vi "校准任务流程.vi"(9 "校准任务":T1[](array[typedef]), 10 "精度":dbl=4.0, 11 "模型":enum32{"线性", "多项式"}(ring)) -> ()   [LabVIEW 2016, in "斯坦道总氮.lvlib"]
uses:
  <userlib>/_OpenG.lib/array/array.llb/Remove Duplicates from 1D Array (U16)__ogtk.vi
panel:
  out "元素":T1
  out "执行列表":T2(ring)
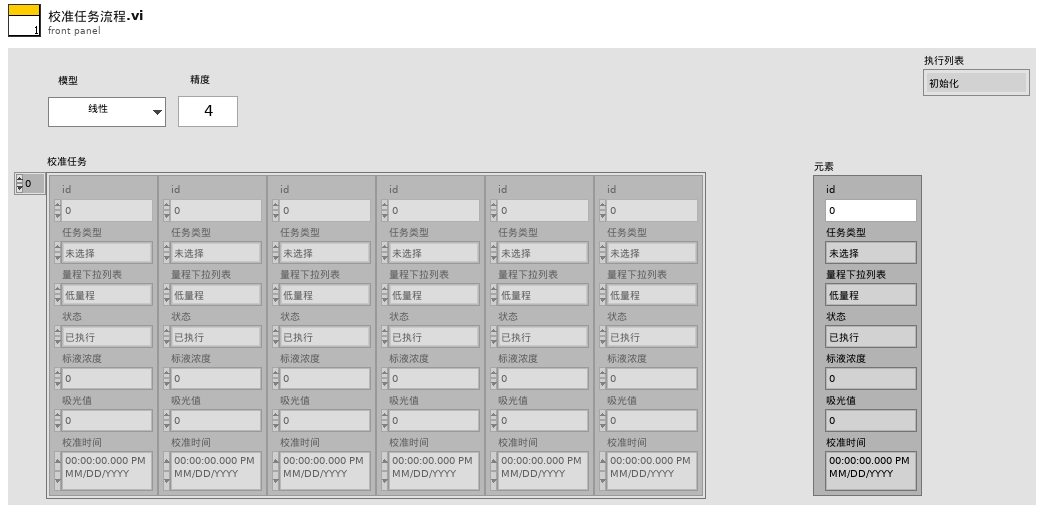
[diagram p1: front panel]
types:
  T1 = typedef "斯坦道总氮.lvlib/校准任务.ctl" = cluster{"id":u16, "任务类型":enum16{"未选择", "空白校准", "标样校准", "标样核查", "零点核查", "跨度核查"}, "量程下拉列表":enum16{"低量程", "高量程"}, "状态":enum16{"已执行", "待执行", "执行中", "停止"}, "标液浓度":dbl, "吸光值":dbl, "校准时间":timestamp}
  T2 = enum16{"初始化", "解析数据", "判断任务类型", "执行测试任务", "等待测试任务完成", "获取测试数据", "任务结束判定", "计算公式", "结束"}
  T3 = cluster{"时间标识":timestamp, "设备":string, "日志信息":string, "流程参数":string}
  T4 = cluster{"站号":u16, "量程切换":enum32{"H", "L", "AUTO"}, "控制命令":enum16{"启动测量", "标样核查", "零点核查", "跨度核查", "空白测试", "平行样测试", "加标回收", "空白校准", "标样校准", "初始化（清洗）", "停止测试", "仪器重启", "校时", "模式设置", "测量间隔设置"}, "模式设置":enum16{"待机", "连续模式", "周期模式", "定点模式", "受控模式", "手动模式"}, "测量间隔":u16}
  T5 = enum16{"启动测量", "标样核查", "零点核查", "跨度核查", "空白测试", "平行样测试", "加标回收", "空白校准", "标样校准", "初始化（清洗）", "停止测试", "仪器重启", "校时", "模式设置", "测量间隔设置"}
  T6 = cluster{"标液浓度1":dbl, "测量吸光度1":dbl, "样品1启用":bool, "标液浓度2":dbl, "测量吸光度2":dbl, "样品2启用":bool, "标液浓度3":dbl, "测量吸光度3":dbl, "样品3启用":bool, "标液浓度4":dbl, "测量吸光度4":dbl, "样品4启用":bool, "标液浓度5":dbl, "测量吸光度5":dbl, "样品5启用":bool, "模型":enum32{"线性", "多项式"}, "精度":dbl, "XY图":cluster{"X Values":dbl[], "Y Values":dbl[]}[], "拟合公式":string, "r^2":dbl, "标样一校准时间":timestamp, "标样二校准时间":timestamp, "标样三校准时间":timestamp, "标样四校准时间":timestamp, "标样五校准时间":timestamp, "二次方程":cluster{"c":dbl, "x":dbl, "x^2":dbl}, "标定时间":timestamp}
  T7 = cluster{"因子编码":u32, "单位":u16, "标样参考值":sgl, "水样数据时间":timestamp, "水样实测值":sgl, "水样数据标识":string, "标样数据时间":timestamp, "标样实测值":sgl, "标样数据标识":string, "空白数据时间":timestamp, "空白实测值":sgl, "空白数据标识":string, "零点核查数据时间":timestamp, "零点核查实测值":sgl, "零点核查数据标识":string, "跨度核查数据时间":timestamp, "跨度核查实测值":sgl, "跨度核查数据标识":string, "加标回收数据时间":timestamp, "加标回收实测值":sgl, "加标回收数据标识":string, "平行样数据时间":timestamp, "平行样实测值":sgl, "平行样数据标识":string, "F0":sgl, "F1":sgl, "F2":sgl, "F3":sgl, "F4":sgl, "F5":sgl, "F6":sgl, "F7":sgl, "温度":sgl, "湿度":sgl, "X值":sgl, "fidrange":u16, "X1值":sgl}
  T8 = cluster{"系统时间":timestamp, "工作状态":u16, "测量模式":enum16{"待机", "连续模式", "周期模式", "定点模式", "受控模式", "手动模式"}, "告警代码":u16, "故障代码":u16, "日志代码":u16, "软件版本":u16, "F0":sgl, "F1":sgl, "F2":sgl, "F3":sgl, "T":sgl, "H":sgl, "id":u16, "flowid":u16, "量程":u16, "总磷控温温度1":sgl, "营养盐控温温度2":sgl, "ADC":sgl, "结果值":sgl, "运行时间":u16, "步骤详情":string, "步骤流程":string}
  T9 = enum16{"未选择", "空白校准", "标样校准", "标样核查", "零点核查", "跨度核查"}
  T10 = cluster{"标液浓度1":dbl, "测量吸光度1":dbl, "样品1启用":bool, "标液浓度2":dbl, "测量吸光度2":dbl, "样品2启用":bool, "标液浓度3":dbl, "测量吸光度3":dbl, "样品3启用":bool, "标液浓度4":dbl, "测量吸光度4":dbl, "样品4启用":bool, "标液浓度5":dbl, "测量吸光度5":dbl, "样品5启用":bool, "模型":enum32{"线性", "多项式"}, "精度":dbl, "XY图":cluster{"X Values":dbl[], "Y Values":dbl[]}[], "拟合公式":string, "r^2":dbl, "标样一校准时间":timestamp, "标样二校准时间":timestamp, "标样三校准时间":timestamp, "标样四校准时间":timestamp, "标样五校准时间":timestamp, "二次方程":cluster{"c":dbl, "x":dbl, "x^2":dbl}, "标定时间":timestamp}[]
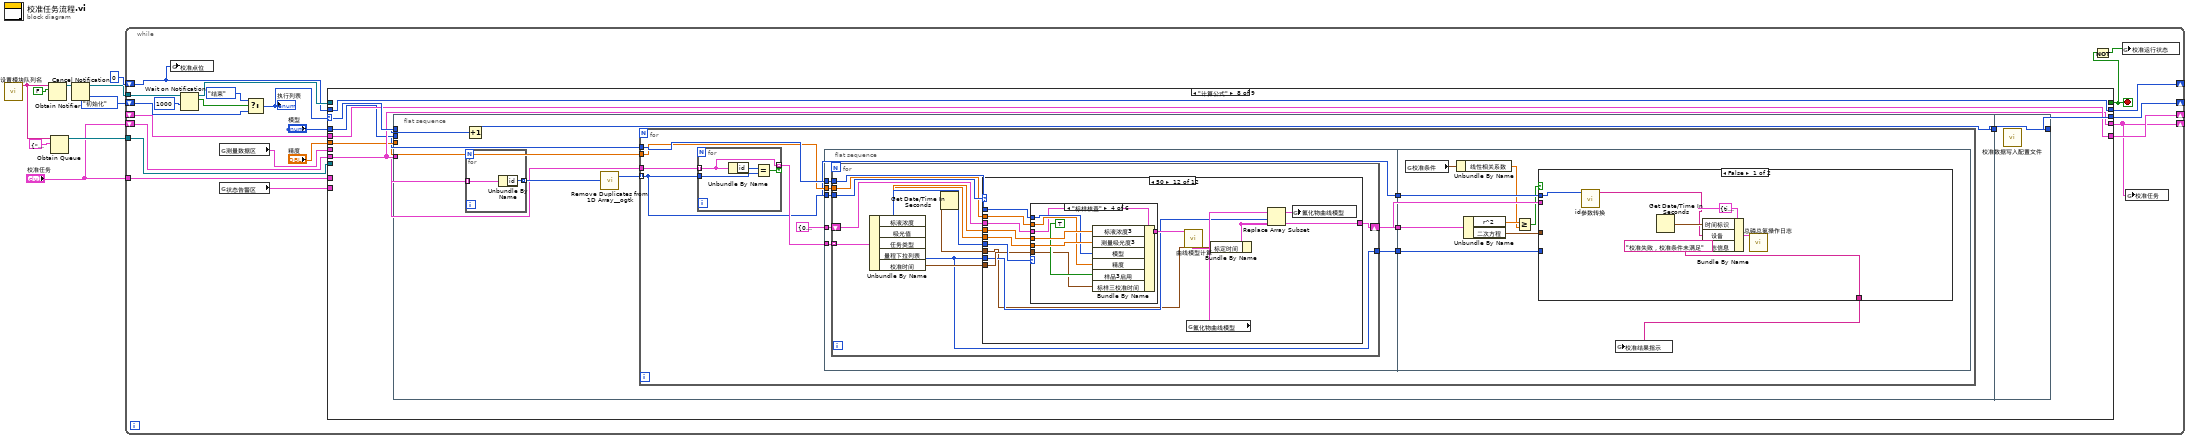
[diagram p0: block diagram]
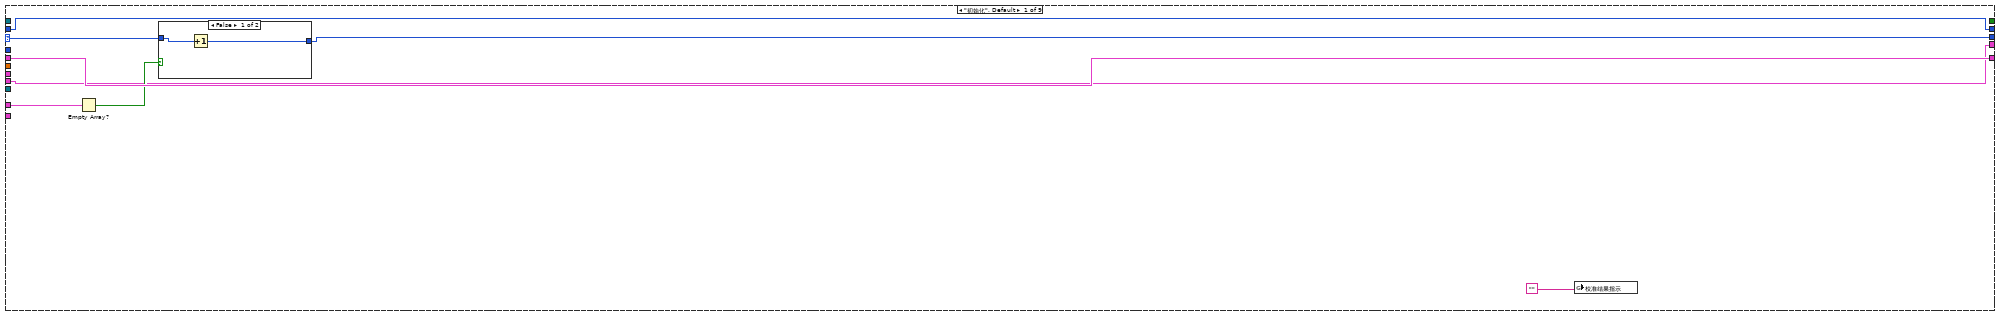
[diagram p2: hidden frame]
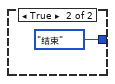
[diagram p3: hidden frame]
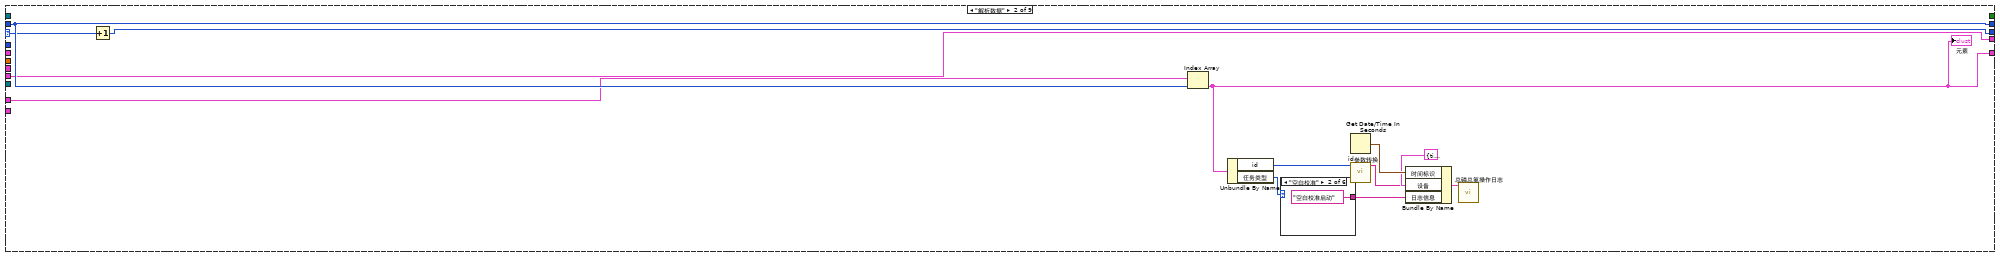
[diagram p4: hidden frame]
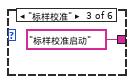
[diagram p6: hidden frame]
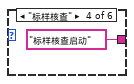
[diagram p7: hidden frame]
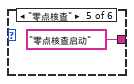
[diagram p8: hidden frame]
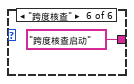
[diagram p9: hidden frame]
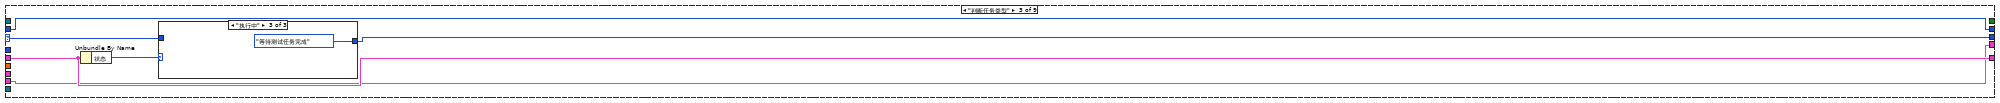
[diagram p10: hidden frame]
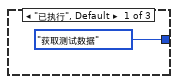
[diagram p11: hidden frame]
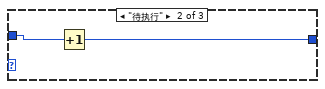
[diagram p12: hidden frame]
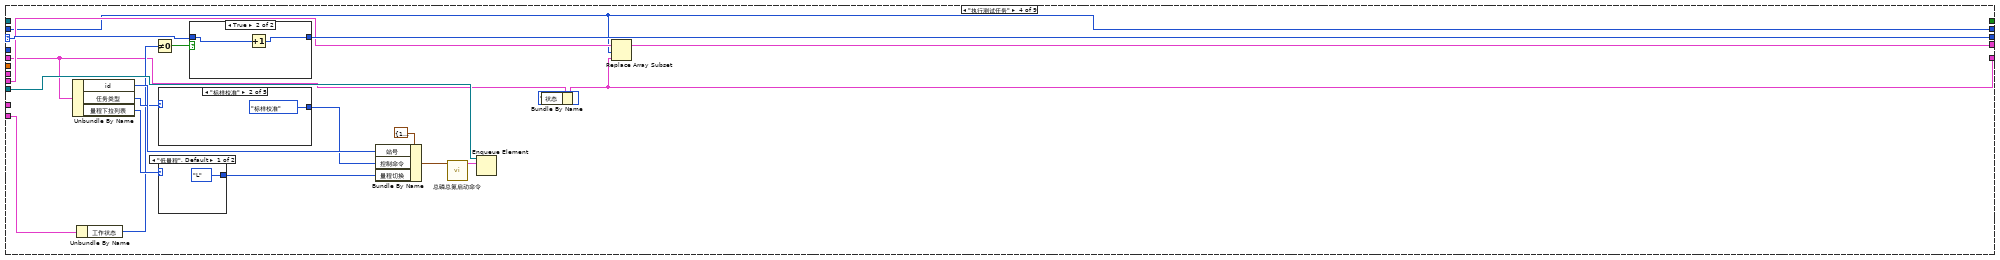
[diagram p13: hidden frame]
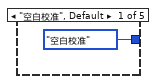
[diagram p15: hidden frame]
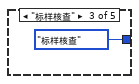
[diagram p16: hidden frame]
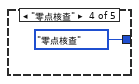
[diagram p17: hidden frame]
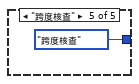
[diagram p18: hidden frame]
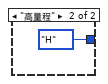
[diagram p19: hidden frame]
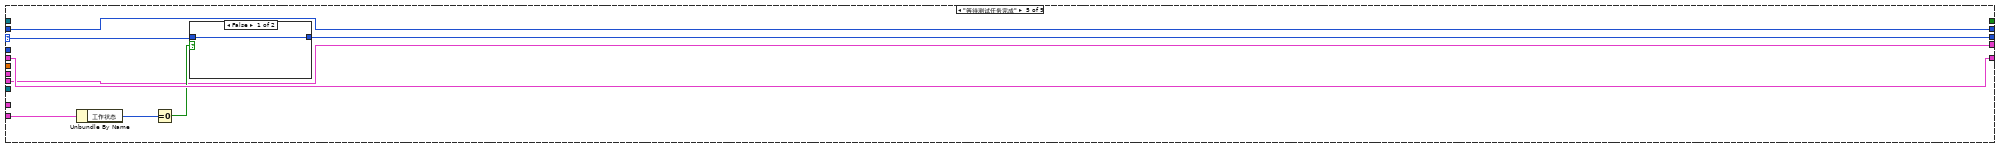
[diagram p20: hidden frame]
diagram:
  n1 = call "设置模块队列名.vi"() -> ("Msg"=w5:string)  [unwired: 5 in]
  n2 = Obtain Notifier(name (unnamed)=w5, notification data type=FALSE) -> (notifier out=w3:refnum<notifier>)  [unwired: 2 in, 2 out]
  n3 = Obtain Queue(name (unnamed)=w5, element data type=cluster{"命令":string, "data":variant} {"命令"="", "data"=variant}) -> (queue out=w4:refnum<queue>)  [unwired: 3 in, 2 out]
  n4 = Cancel Notification(0:w3) -> (8:w2:refnum<notifier>)  [unwired: 1 in, 2 out]
  n5 = while {
    shift-right: [w29] -> _
    shift-left: 0 -> [w11]
    shift-right: [w31] -> _
    shift-left: _ -> [w30]
    shift-right: [w28] -> _
    shift-left: T2."初始化" ("执行列表") -> [w17]
    tunnel: w4 -> [w27]
    tunnel: w2 -> [w26]
    tunnel: "校准任务" -> [w23]
    shift-right: [w10] -> _
    shift-left: "校准任务" -> [w22]
    stop <- w12 stop-if-true
    n6 = global write "VAR总磷总氮全局变量.vi" "校准点位"(w11) -> ()
    n7 = Wait on Notification(notifier=w26, timeout in ms (-1)=1000 ("超时毫秒(-1)")) -> (notifier out=w19:refnum<notifier>, notification=w18:bool)  [unwired: 2 in, 2 out]
    n8 = global read "VAR总磷总氮全局变量.vi" "测量数据区"() -> (w24:T7)
    n9 = global read "VAR总磷总氮全局变量.vi" "状态告警区"() -> (w25:T8)
    n10 = Select(t=T2."结束", s=w18, f=w17) -> (s? t:f=w16:T2)
    "执行列表" <- w16
    n11 = case shown="\"计算公式\"" w16 {
      selector: w16 -> [w37 w54 w63 w78 w104 w121 w152 w165 w859]
      tunnel: w11 -> [w38 w55 w65 w74 w107 w112 w153 w163 w857]
      tunnel: [w39 w46 w66 w71 w108 w116 w154 w162 w858] -> w31
      tunnel: w30 -> [w39 _ w66 w73 w108 w116 w154 w162 w858]
      tunnel: [w38 w55 w65 w74 w107 w112 w149 w163 w857] -> w29
      tunnel: [_ _ _ _ _ _ _ _ TRUE] -> w12
      tunnel: [w36 w53 w62 w77 w102 w120 w151 w164 w859] -> w28
      tunnel: w27 -> [_ _ _ w89 _ _ _ _ w854]
      tunnel: w19 -> [_ _ _ _ _ _ _ _ w853]
      tunnel: w25 -> [_ _ _ w81 w106 _ _ _ _]
      tunnel: w24 -> [_ _ _ _ _ w123 _ _ _]
      tunnel: w23 -> [w34 w52 _ _ _ _ w150 _ _]
      tunnel: [w33 w51 w61 w75 w101 w118 w146 w161 w855] -> w10
      tunnel: w22 -> [w33 w51 w61 w76 w101 w117 w146 w161 w855]
      tunnel: "模型" -> [_ _ _ _ _ _ _ w160 _]
      tunnel: "精度" -> [_ _ _ _ _ _ _ w159 _]
      frame "初始化", Default {
        n12 = Empty Array?(array=w34) -> (empty?=w35:bool)
        n13 = case shown="False" w35 {
          tunnel: w37 -> [w41 _]
          tunnel: [w40 T2."结束"] -> w36
          frame False {
            n14 = Increment(x=w41) -> (x+1=w40:T2)
          }
          frame True {
          }
        }
        n15 = global write "VAR总磷总氮全局变量.vi" "校准结果指示"("") -> ()
      }
      frame "解析数据" {
        n16 = Increment(x=w54) -> (x+1=w53:T2)
        n17 = Index Array(array=w52, index=w55) -> (element=w46:T1)
        "元素" <- w46
        n18 = Unbundle By Name(w46) -> ("id"=w45:u16, "任务类型"=w44:T9)
        n19 = case shown="\"空白校准\"" w44 {
          tunnel: [_ "空白校准启动" "标样校准启动" "标样核查启动" "零点核查启动" "跨度核查启动"] -> w43
          frame "未选择", Default {
          }
          frame "空白校准" {
          }
          frame "标样校准" {
          }
          frame "标样核查" {
          }
          frame "零点核查" {
          }
          frame "跨度核查" {
          }
        }
        n20 = Get Date/Time In Seconds() -> (seconds since 1Jan1904=w50:timestamp)
        n21 = call "id参数转换.vi"("id"=w45) -> ("table输出"=w47:string)  [unwired: 9 in, 1 out]
        n22 = Bundle By Name(cluster=T3 {"时间标识"=timestamp(0 s since 1904-01-01), "设备"="", "日志信息"="", "流程参数"=""} ("data in"), "时间标识"=w50, "设备"=w47, "日志信息"=w43) -> (w49:T3)
        n23 = call "总磷总氮操作日志.vi"("data in"=w49) -> ()  [unwired: 10 in, 1 out]
      }
      frame "判断任务类型" {
        n24 = Unbundle By Name(w66) -> ("状态"=w64:enum16{"已执行", "待执行", "执行中", "停止"})
        n25 = case shown="\"执行中\"" w64 {
          tunnel: w63 -> [_ w69 _]
          tunnel: [T2."获取测试数据" w68 T2."等待测试任务完成"] -> w62
          frame "已执行", Default {
          }
          frame "待执行" {
            n26 = Increment(x=w69) -> (x+1=w68:T2)
          }
          frame "执行中" {
          }
        }
      }
      frame "执行测试任务" {
        n27 = Unbundle By Name(w73) -> ("id"=w87:u16, "任务类型"=w86:T9, "量程下拉列表"=w85:enum16{"低量程", "高量程"})
        n28 = Unbundle By Name(w81) -> ("工作状态"=w80:u16)
        n29 = Not Equal To 0?(x=w80) -> (x != 0?=w79:bool)
        n30 = case shown="\"标样校准\"" w86 {
          tunnel: [T5."空白校准" ("控制命令") T5."标样校准" ("控制命令") T5."标样核查" ("控制命令") T5."零点核查" ("控制命令") T5."跨度核查" ("控制命令")] -> w84
          frame "空白校准", Default {
          }
          frame "标样校准" {
          }
          frame "标样核查" {
          }
          frame "零点核查" {
          }
          frame "跨度核查" {
          }
        }
        n31 = case shown="\"低量程\", Default" w85 {
          tunnel: [enum32{"H", "L", "AUTO"}."L" ("量程切换") enum32{"H", "L", "AUTO"}."H" ("量程切换")] -> w82
          frame "低量程", Default {
          }
          frame "高量程" {
          }
        }
        n32 = case shown="True" w79 {
          tunnel: w78 -> [w91 w93]
          tunnel: [w91 w92] -> w77
          frame False {
          }
          frame True {
            n33 = Increment(x=w93) -> (x+1=w92:T2)
          }
        }
        n34 = Bundle By Name(cluster=T4 {"站号"=1, "量程切换"=enum."AUTO", "控制命令"=enum."启动测量", "模式设置"=enum."待机", "测量间隔"=0} ("参数"), "站号"=w87, "控制命令"=w84, "量程切换"=w82) -> (w83:T4)
        n35 = call "总磷总氮启动命令.vi"("参数"=w83) -> ("启动命令"=w90:cluster{"命令":string, "data":variant})  [unwired: 10 in]
        n36 = Enqueue Element(queue=w89, element=w90) -> ()  [unwired: 2 in, 3 out]
        n37 = Bundle By Name(cluster=w73, "状态"=enum16{"已执行", "待执行", "执行中", "停止"}."执行中") -> (w71:T1)
        n38 = Replace Array Subset(array=w76, new element=w71, index=w74) -> (w75:T1[])
      }
      frame "等待测试任务完成" {
        n39 = Unbundle By Name(w106) -> ("工作状态"=w105:u16)
        n40 = Equal To 0?(x=w105) -> (x = 0?=w103:bool)
        n41 = case shown="False" w103 {
          tunnel: w104 -> [w109 w111]
          tunnel: [w109 w110] -> w102
          frame False {
          }
          frame True {
            n42 = Increment(x=w111) -> (x+1=w110:T2)
          }
        }
      }
      frame "获取测试数据" {
        n43 = Unbundle By Name(w116) -> ("任务类型"=w122:T9, "状态"=w115:enum16{"已执行", "待执行", "执行中", "停止"})
        n44 = Increment(x=w121) -> (x+1=w120:T2)
        n45 = case shown="\"已执行\", Default" w115 {
          tunnel: w123 -> [_ w130]
          tunnel: w122 -> [_ w129]
          tunnel: [w124 w126] -> w119
          tunnel: w116 -> [w124 w125]
          frame "已执行", Default {
          }
          frame "执行中" {
            n46 = case shown="\"标样校准\"" w129 {
              tunnel: w130 -> [w133 w136 w139 w142 w145]
              tunnel: [w132 w135 w138 w141 w144] -> w127
              tunnel: [w131 w134 w137 w140 w143] -> w128
              frame "空白校准", Default {
                n47 = Unbundle By Name(w133) -> ("空白数据时间"=w132:timestamp, "X值"=w131:sgl)
              }
              frame "标样校准" {
                n48 = Unbundle By Name(w136) -> ("标样数据时间"=w135:timestamp, "X值"=w134:sgl)
              }
              frame "标样核查" {
                n49 = Unbundle By Name(w139) -> ("标样数据时间"=w138:timestamp, "X值"=w137:sgl)
              }
              frame "零点核查" {
                n50 = Unbundle By Name(w142) -> ("零点核查数据时间"=w141:timestamp, "X值"=w140:sgl)
              }
              frame "跨度核查" {
                n51 = Unbundle By Name(w145) -> ("跨度核查数据时间"=w144:timestamp, "X值"=w143:sgl)
              }
            }
            n52 = Bundle By Name(cluster=w125, "校准时间"=w127, "吸光值"=w128) -> (w126:T1)
          }
        }
        n53 = Bundle By Name(cluster=w119, "状态"=enum16{"已执行", "待执行", "执行中", "停止"}."已执行") -> (w113:T1)
        n54 = Replace Array Subset(array=w117, new element=w113, index=w112) -> (w118:T1[])
      }
      frame "任务结束判定" {
        n55 = Array Size(array=w150) -> (size(s)=w148:i32)
        n56 = Increment(x=w153) -> (x+1=w149:i32)
        n57 = Greater Or Equal?(x=w149, y=w148) -> (x >= y?=w147:bool)
        n58 = case shown="False" w147 {
          tunnel: w152 -> [_ w157]
          tunnel: [T2."解析数据" w156] -> w151
          frame False {
          }
          frame True {
            n59 = Increment(x=w157) -> (x+1=w156:T2)
          }
        }
      }
      frame "计算公式" {
        n60 = flat-sequence {
          tunnel: w165 -> [w172]
          tunnel: w161 -> [w168]
          tunnel: w160 -> [w167]
          tunnel: w159 -> [w166]
          tunnel: [w171] -> w158
          tunnel: [w852] -> w164
          tunnel: w158 -> [w852]
          frame #0 {
            n61 = for {
              tunnel: w168 -> [w851] mode=indexing
              tunnel: [w850] -> w170 mode=indexing
              n62 = Unbundle By Name(w851) -> ("id"=w850:u16)
            }
            n63 = Increment(x=w172) -> (x+1=w171:T2)
            n64 = call-poly <userlib>:"Remove Duplicates from 1D Array__ogtk.vi"("Input Array"=w170) -> ("Output Array"=w169:u16[])  [unwired: 1 out]
            n65 = for {
              tunnel: w169 -> [w179] mode=indexing
              tunnel: w168 -> [w181]
              tunnel: w167 -> [w178]
              tunnel: w166 -> [w177]
              n66 = for {
                tunnel: w181 -> [w847] mode=indexing
                tunnel: w179 -> [w849]
                tunnel: [w847] -> w180 mode=indexing if=w848
                n67 = Unbundle By Name(w847) -> ("id"=w846:u16)
                n68 = Equal?(x=w846, y=w849) -> (x = y?=w848:bool)
              }
              n69 = flat-sequence {
                tunnel: w180 -> [w188]
                tunnel: w179 -> [w183]
                tunnel: w178 -> [w187]
                tunnel: w177 -> [w186]
                tunnel: T6 {"标液浓度1"=0.0, "测量吸光度1"=0.0, "样品1启用"=FALSE, "标液浓度2"=0.0, "测量吸光度2"=0.0, "样品2启用"=FALSE, "标液浓度3"=0.0, "测量吸光度3"=0.0, "样品3启用"=FALSE, "标液浓度4"=0.0, "测量吸光度4"=0.0, "样品4启用"=FALSE, "标液浓度5"=0.0, "测量吸光度5"=0.0, "样品5启用"=FALSE, "模型"=enum."线性", "精度"=0.0, "XY图"=[], "拟合公式"="", "r^2"=0.0, "标样一校准时间"=timestamp(0 s since 1904-01-01), "标样二校准时间"=timestamp(0 s since 1904-01-01), "标样三校准时间"=timestamp(0 s since 1904-01-01), "标样四校准时间"=timestamp(0 s since 1904-01-01), "标样五校准时间"=timestamp(0 s since 1904-01-01), "二次方程"={"c"=0.0, "x"=0.0, "x^2"=0.0}, "标定时间"=timestamp(0 s since 1904-01-01)} ("新元素/子数组") -> [w185]
                tunnel: [w184] -> w175
                tunnel: [w183] -> w174
                tunnel: [w182] -> w173
                tunnel: w175 -> [w812]
                tunnel: w174 -> [w814]
                tunnel: w173 -> [w813]
                frame #0 {
                  n70 = for {
                    tunnel: w188 -> [w200] mode=indexing
                    tunnel: w183 -> [w199]
                    tunnel: w187 -> [w195]
                    tunnel: w186 -> [w194]
                    shift-right: [w192] -> w184
                    shift-left: w185 -> [w193]
                    tunnel: [w190] -> w182
                    n71 = Unbundle By Name(w200) -> ("标液浓度"=w197:dbl, "吸光值"=w196:dbl, "任务类型"=w198:T9, "量程下拉列表"=w190:enum16{"低量程", "高量程"}, "校准时间"=w191:timestamp)
                    n72 = Get Date/Time In Seconds() -> (seconds since 1Jan1904=w189:timestamp)
                    n73 = case shown="50" w199 {
                      tunnel: w190 -> [_ w204 w261 w316 w372 w425 w479 w535 w591 w645 w700 w755]
                      tunnel: w198 -> [_ w215 w270 w325 w380 w435 w490 w545 w600 w655 w710 w765]
                      tunnel: w197 -> [_ w214 w269 w324 w379 w434 w489 w544 w599 w654 w709 w764]
                      tunnel: w196 -> [_ w213 w268 w323 w378 w433 w488 w543 w598 w653 w708 w763]
                      tunnel: w195 -> [_ w212 w267 w322 w377 w432 w487 w542 w597 w652 w707 w762]
                      tunnel: w194 -> [_ w211 w266 w321 w376 w431 w486 w541 w596 w651 w706 w761]
                      tunnel: w193 -> [w201 w210 w265 w320 w375 w430 w485 w540 w595 w650 w705 w760]
                      tunnel: [w201 w203 w258 w313 w368 w423 w478 w533 w588 w643 w698 w753] -> w192
                      tunnel: w191 -> [_ w209 w264 w319 w374 w429 w484 w539 w594 w649 w704 w759]
                      tunnel: w189 -> [_ w202 w257 w312 w367 w422 w477 w532 w587 w642 w697 w752]
                      frame 0, Default {
                      }
                      frame 1 {
                        n74 = case shown="\"未选择\", Default" w215 {
                          tunnel: w214 -> [_ w224 w232 w240 w248 w256]
                          tunnel: w213 -> [_ w223 w231 w239 w247 w255]
                          tunnel: w212 -> [_ w222 w230 w238 w246 w254]
                          tunnel: w211 -> [_ w221 w229 w237 w245 w253]
                          tunnel: w210 -> [w216 w219 w227 w235 w243 w251]
                          tunnel: [w216 w217 w226 w234 w242 w250] -> w206
                          tunnel: w209 -> [_ w218 w225 w233 w241 w249]
                          frame "未选择", Default {
                          }
                          frame "空白校准" {
                            n75 = Bundle By Name(cluster=w219, "标液浓度1"=w224, "测量吸光度1"=w223, "模型"=w222, "精度"=w221, "样品1启用"=TRUE, "标样一校准时间"=w218) -> (w217:T6)
                          }
                          frame "标样校准" {
                            n76 = Bundle By Name(cluster=w227, "标液浓度2"=w232, "测量吸光度2"=w231, "模型"=w230, "精度"=w229, "样品2启用"=TRUE ("样品1启用"), "标样二校准时间"=w225) -> (w226:T6)
                          }
                          frame "标样核查" {
                            n77 = Bundle By Name(cluster=w235, "标液浓度3"=w240, "测量吸光度3"=w239, "模型"=w238, "精度"=w237, "样品3启用"=TRUE ("样品1启用"), "标样三校准时间"=w233) -> (w234:T6)
                          }
                          frame "零点核查" {
                            n78 = Bundle By Name(cluster=w243, "标液浓度4"=w248, "测量吸光度4"=w247, "模型"=w246, "精度"=w245, "样品4启用"=TRUE ("样品1启用"), "标样四校准时间"=w241) -> (w242:T6)
                          }
                          frame "跨度核查" {
                            n79 = Bundle By Name(cluster=w251, "标液浓度5"=w256, "测量吸光度5"=w255, "模型"=w254, "精度"=w253, "样品5启用"=TRUE ("样品1启用"), "标样五校准时间"=w249) -> (w250:T6)
                          }
                        }
                        n80 = call "曲线模型计算.vi"("曲线模型"=w206) -> ("输出簇"=w205:T6)  [unwired: 10 in]
                        n81 = global read "校准数据全局变量.vi" "总磷曲线模型"() -> (w208:T10)
                        n82 = Bundle By Name(cluster=w205, "标定时间"=w202) -> (w203:T6)
                        n83 = Replace Array Subset(array=w208, new element=w203, index=w204) -> (w207:T10)
                        n84 = global write "校准数据全局变量.vi" "总磷曲线模型"(w207) -> ()
                      }
                      frame 2 {
                        n85 = case shown="\"标样校准\"" w270 {
                          tunnel: w269 -> [_ w279 w287 w295 w303 w311]
                          tunnel: w268 -> [_ w278 w286 w294 w302 w310]
                          tunnel: w267 -> [_ w277 w285 w293 w301 w309]
                          tunnel: w266 -> [_ w276 w284 w292 w300 w308]
                          tunnel: w265 -> [w271 w274 w282 w290 w298 w306]
                          tunnel: [w271 w273 w281 w289 w297 w305] -> w263
                          tunnel: w264 -> [_ w272 w280 w288 w296 w304]
                          frame "未选择", Default {
                          }
                          frame "空白校准" {
                            n86 = Bundle By Name(cluster=w274, "标液浓度1"=w279, "测量吸光度1"=w278, "模型"=w277, "精度"=w276, "样品1启用"=TRUE, "标样一校准时间"=w272) -> (w273:T6)
                          }
                          frame "标样校准" {
                            n87 = Bundle By Name(cluster=w282, "标液浓度2"=w287, "测量吸光度2"=w286, "模型"=w285, "精度"=w284, "样品2启用"=TRUE ("样品1启用"), "标样二校准时间"=w280) -> (w281:T6)
                          }
                          frame "标样核查" {
                            n88 = Bundle By Name(cluster=w290, "标液浓度3"=w295, "测量吸光度3"=w294, "模型"=w293, "精度"=w292, "样品3启用"=TRUE ("样品1启用"), "标样三校准时间"=w288) -> (w289:T6)
                          }
                          frame "零点核查" {
                            n89 = Bundle By Name(cluster=w298, "标液浓度4"=w303, "测量吸光度4"=w302, "模型"=w301, "精度"=w300, "样品4启用"=TRUE ("样品1启用"), "标样四校准时间"=w296) -> (w297:T6)
                          }
                          frame "跨度核查" {
                            n90 = Bundle By Name(cluster=w306, "标液浓度5"=w311, "测量吸光度5"=w310, "模型"=w309, "精度"=w308, "样品5启用"=TRUE ("样品1启用"), "标样五校准时间"=w304) -> (w305:T6)
                          }
                        }
                        n91 = call "曲线模型计算.vi"("曲线模型"=w263) -> ("输出簇"=w259:T6)  [unwired: 10 in]
                        n92 = global read "校准数据全局变量.vi" "总氮曲线模型"() -> (w262:T10)
                        n93 = Bundle By Name(cluster=w259, "标定时间"=w257) -> (w258:T6)
                        n94 = Replace Array Subset(array=w262, new element=w258, index=w261) -> (w260:T10)
                        n95 = global write "校准数据全局变量.vi" "总氮曲线模型"(w260) -> ()
                      }
                      frame 3 {
                        n96 = case shown="\"标样校准\"" w325 {
                          tunnel: w324 -> [_ w334 w342 w350 w358 w366]
                          tunnel: w323 -> [_ w333 w341 w349 w357 w365]
                          tunnel: w322 -> [_ w332 w340 w348 w356 w364]
                          tunnel: w321 -> [_ w331 w339 w347 w355 w363]
                          tunnel: w320 -> [w326 w329 w337 w345 w353 w361]
                          tunnel: [w326 w328 w336 w344 w352 w360] -> w315
                          tunnel: w319 -> [_ w327 w335 w343 w351 w359]
                          frame "未选择", Default {
                          }
                          frame "空白校准" {
                            n97 = Bundle By Name(cluster=w329, "标液浓度1"=w334, "测量吸光度1"=w333, "模型"=w332, "精度"=w331, "样品1启用"=TRUE, "标样一校准时间"=w327) -> (w328:T6)
                          }
                          frame "标样校准" {
                            n98 = Bundle By Name(cluster=w337, "标液浓度2"=w342, "测量吸光度2"=w341, "模型"=w340, "精度"=w339, "样品2启用"=TRUE ("样品1启用"), "标样二校准时间"=w335) -> (w336:T6)
                          }
                          frame "标样核查" {
                            n99 = Bundle By Name(cluster=w345, "标液浓度3"=w350, "测量吸光度3"=w349, "模型"=w348, "精度"=w347, "样品3启用"=TRUE ("样品1启用"), "标样三校准时间"=w343) -> (w344:T6)
                          }
                          frame "零点核查" {
                            n100 = Bundle By Name(cluster=w353, "标液浓度4"=w358, "测量吸光度4"=w357, "模型"=w356, "精度"=w355, "样品4启用"=TRUE ("样品1启用"), "标样四校准时间"=w351) -> (w352:T6)
                          }
                          frame "跨度核查" {
                            n101 = Bundle By Name(cluster=w361, "标液浓度5"=w366, "测量吸光度5"=w365, "模型"=w364, "精度"=w363, "样品5启用"=TRUE ("样品1启用"), "标样五校准时间"=w359) -> (w360:T6)
                          }
                        }
                        n102 = call "曲线模型计算.vi"("曲线模型"=w315) -> ("输出簇"=w314:T6)  [unwired: 10 in]
                        n103 = global read "校准数据全局变量.vi" "氨氮曲线模型"() -> (w318:T10)
                        n104 = Bundle By Name(cluster=w314, "标定时间"=w312) -> (w313:T6)
                        n105 = Replace Array Subset(array=w318, new element=w313, index=w316) -> (w317:T10)
                        n106 = global write "校准数据全局变量.vi" "氨氮曲线模型"(w317) -> ()
                      }
                      frame 4 {
                        n107 = case shown="\"空白校准\"" w380 {
                          tunnel: w379 -> [_ w389 w397 w405 w413 w421]
                          tunnel: w378 -> [_ w388 w396 w404 w412 w420]
                          tunnel: w377 -> [_ w387 w395 w403 w411 w419]
                          tunnel: w376 -> [_ w386 w394 w402 w410 w418]
                          tunnel: w375 -> [w381 w384 w392 w400 w408 w416]
                          tunnel: [w381 w383 w391 w399 w407 w415] -> w371
                          tunnel: w374 -> [_ w382 w390 w398 w406 w414]
                          frame "未选择", Default {
                          }
                          frame "空白校准" {
                            n108 = Bundle By Name(cluster=w384, "标液浓度1"=w389, "测量吸光度1"=w388, "模型"=w387, "精度"=w386, "样品1启用"=TRUE, "标样一校准时间"=w382) -> (w383:T6)
                          }
                          frame "标样校准" {
                            n109 = Bundle By Name(cluster=w392, "标液浓度2"=w397, "测量吸光度2"=w396, "模型"=w395, "精度"=w394, "样品2启用"=TRUE ("样品1启用"), "标样二校准时间"=w390) -> (w391:T6)
                          }
                          frame "标样核查" {
                            n110 = Bundle By Name(cluster=w400, "标液浓度3"=w405, "测量吸光度3"=w404, "模型"=w403, "精度"=w402, "样品3启用"=TRUE ("样品1启用"), "标样三校准时间"=w398) -> (w399:T6)
                          }
                          frame "零点核查" {
                            n111 = Bundle By Name(cluster=w408, "标液浓度4"=w413, "测量吸光度4"=w412, "模型"=w411, "精度"=w410, "样品4启用"=TRUE ("样品1启用"), "标样四校准时间"=w406) -> (w407:T6)
                          }
                          frame "跨度核查" {
                            n112 = Bundle By Name(cluster=w416, "标液浓度5"=w421, "测量吸光度5"=w420, "模型"=w419, "精度"=w418, "样品5启用"=TRUE ("样品1启用"), "标样五校准时间"=w414) -> (w415:T6)
                          }
                        }
                        n113 = call "曲线模型计算.vi"("曲线模型"=w371) -> ("输出簇"=w369:T6)  [unwired: 10 in]
                        n114 = global read "校准数据全局变量.vi" "磷酸盐曲线模型"() -> (w373:T10)
                        n115 = Bundle By Name(cluster=w369, "标定时间"=w367) -> (w368:T6)
                        n116 = Replace Array Subset(array=w373, new element=w368, index=w372) -> (w370:T10)
                        n117 = global write "校准数据全局变量.vi" "磷酸盐曲线模型"(w370) -> ()
                      }
                      frame 5 {
                        n118 = case shown="\"跨度核查\"" w435 {
                          tunnel: w434 -> [_ w444 w452 w460 w468 w476]
                          tunnel: w433 -> [_ w443 w451 w459 w467 w475]
                          tunnel: w432 -> [_ w442 w450 w458 w466 w474]
                          tunnel: w431 -> [_ w441 w449 w457 w465 w473]
                          tunnel: w430 -> [w436 w439 w447 w455 w463 w471]
                          tunnel: [w436 w438 w446 w454 w462 w470] -> w428
                          tunnel: w429 -> [_ w437 w445 w453 w461 w469]
                          frame "未选择", Default {
                          }
                          frame "空白校准" {
                            n119 = Bundle By Name(cluster=w439, "标液浓度1"=w444, "测量吸光度1"=w443, "模型"=w442, "精度"=w441, "样品1启用"=TRUE, "标样一校准时间"=w437) -> (w438:T6)
                          }
                          frame "标样校准" {
                            n120 = Bundle By Name(cluster=w447, "标液浓度2"=w452, "测量吸光度2"=w451, "模型"=w450, "精度"=w449, "样品2启用"=TRUE ("样品1启用"), "标样二校准时间"=w445) -> (w446:T6)
                          }
                          frame "标样核查" {
                            n121 = Bundle By Name(cluster=w455, "标液浓度3"=w460, "测量吸光度3"=w459, "模型"=w458, "精度"=w457, "样品3启用"=TRUE ("样品1启用"), "标样三校准时间"=w453) -> (w454:T6)
                          }
                          frame "零点核查" {
                            n122 = Bundle By Name(cluster=w463, "标液浓度4"=w468, "测量吸光度4"=w467, "模型"=w466, "精度"=w465, "样品4启用"=TRUE ("样品1启用"), "标样四校准时间"=w461) -> (w462:T6)
                          }
                          frame "跨度核查" {
                            n123 = Bundle By Name(cluster=w471, "标液浓度5"=w476, "测量吸光度5"=w475, "模型"=w474, "精度"=w473, "样品5启用"=TRUE ("样品1启用"), "标样五校准时间"=w469) -> (w470:T6)
                          }
                        }
                        n124 = call "曲线模型计算.vi"("曲线模型"=w428) -> ("输出簇"=w426:T6)  [unwired: 10 in]
                        n125 = global read "校准数据全局变量.vi" "硝氮曲线模型"() -> (w427:T10)
                        n126 = Bundle By Name(cluster=w426, "标定时间"=w422) -> (w423:T6)
                        n127 = Replace Array Subset(array=w427, new element=w423, index=w425) -> (w424:T10)
                        n128 = global write "校准数据全局变量.vi" "硝氮曲线模型"(w424) -> ()
                      }
                      frame 6 {
                        n129 = case shown="\"标样校准\"" w490 {
                          tunnel: w489 -> [_ w499 w507 w515 w523 w531]
                          tunnel: w488 -> [_ w498 w506 w514 w522 w530]
                          tunnel: w487 -> [_ w497 w505 w513 w521 w529]
                          tunnel: w486 -> [_ w496 w504 w512 w520 w528]
                          tunnel: w485 -> [w491 w494 w502 w510 w518 w526]
                          tunnel: [w491 w493 w501 w509 w517 w525] -> w481
                          tunnel: w484 -> [_ w492 w500 w508 w516 w524]
                          frame "未选择", Default {
                          }
                          frame "空白校准" {
                            n130 = Bundle By Name(cluster=w494, "标液浓度1"=w499, "测量吸光度1"=w498, "模型"=w497, "精度"=w496, "样品1启用"=TRUE, "标样一校准时间"=w492) -> (w493:T6)
                          }
                          frame "标样校准" {
                            n131 = Bundle By Name(cluster=w502, "标液浓度2"=w507, "测量吸光度2"=w506, "模型"=w505, "精度"=w504, "样品2启用"=TRUE ("样品1启用"), "标样二校准时间"=w500) -> (w501:T6)
                          }
                          frame "标样核查" {
                            n132 = Bundle By Name(cluster=w510, "标液浓度3"=w515, "测量吸光度3"=w514, "模型"=w513, "精度"=w512, "样品3启用"=TRUE ("样品1启用"), "标样三校准时间"=w508) -> (w509:T6)
                          }
                          frame "零点核查" {
                            n133 = Bundle By Name(cluster=w518, "标液浓度4"=w523, "测量吸光度4"=w522, "模型"=w521, "精度"=w520, "样品4启用"=TRUE ("样品1启用"), "标样四校准时间"=w516) -> (w517:T6)
                          }
                          frame "跨度核查" {
                            n134 = Bundle By Name(cluster=w526, "标液浓度5"=w531, "测量吸光度5"=w530, "模型"=w529, "精度"=w528, "样品5启用"=TRUE ("样品1启用"), "标样五校准时间"=w524) -> (w525:T6)
                          }
                        }
                        n135 = call "曲线模型计算.vi"("曲线模型"=w481) -> ("输出簇"=w480:T6)  [unwired: 10 in]
                        n136 = global read "校准数据全局变量.vi" "亚硝氮曲线模型"() -> (w483:T10)
                        n137 = Bundle By Name(cluster=w480, "标定时间"=w477) -> (w478:T6)
                        n138 = Replace Array Subset(array=w483, new element=w478, index=w479) -> (w482:T10)
                        n139 = global write "校准数据全局变量.vi" "亚硝氮曲线模型"(w482) -> ()
                      }
                      frame 7 {
                        n140 = case shown="\"未选择\", Default" w545 {
                          tunnel: w544 -> [_ w554 w562 w570 w578 w586]
                          tunnel: w543 -> [_ w553 w561 w569 w577 w585]
                          tunnel: w542 -> [_ w552 w560 w568 w576 w584]
                          tunnel: w541 -> [_ w551 w559 w567 w575 w583]
                          tunnel: w540 -> [w546 w549 w557 w565 w573 w581]
                          tunnel: [w546 w548 w556 w564 w572 w580] -> w538
                          tunnel: w539 -> [_ w547 w555 w563 w571 w579]
                          frame "未选择", Default {
                          }
                          frame "空白校准" {
                            n141 = Bundle By Name(cluster=w549, "标液浓度1"=w554, "测量吸光度1"=w553, "模型"=w552, "精度"=w551, "样品1启用"=TRUE, "标样一校准时间"=w547) -> (w548:T6)
                          }
                          frame "标样校准" {
                            n142 = Bundle By Name(cluster=w557, "标液浓度2"=w562, "测量吸光度2"=w561, "模型"=w560, "精度"=w559, "样品2启用"=TRUE ("样品1启用"), "标样二校准时间"=w555) -> (w556:T6)
                          }
                          frame "标样核查" {
                            n143 = Bundle By Name(cluster=w565, "标液浓度3"=w570, "测量吸光度3"=w569, "模型"=w568, "精度"=w567, "样品3启用"=TRUE ("样品1启用"), "标样三校准时间"=w563) -> (w564:T6)
                          }
                          frame "零点核查" {
                            n144 = Bundle By Name(cluster=w573, "标液浓度4"=w578, "测量吸光度4"=w577, "模型"=w576, "精度"=w575, "样品4启用"=TRUE ("样品1启用"), "标样四校准时间"=w571) -> (w572:T6)
                          }
                          frame "跨度核查" {
                            n145 = Bundle By Name(cluster=w581, "标液浓度5"=w586, "测量吸光度5"=w585, "模型"=w584, "精度"=w583, "样品5启用"=TRUE ("样品1启用"), "标样五校准时间"=w579) -> (w580:T6)
                          }
                        }
                        n146 = call "曲线模型计算.vi"("曲线模型"=w538) -> ("输出簇"=w536:T6)  [unwired: 10 in]
                        n147 = global read "校准数据全局变量.vi" "硅酸盐曲线模型"() -> (w537:T10)
                        n148 = Bundle By Name(cluster=w536, "标定时间"=w532) -> (w533:T6)
                        n149 = Replace Array Subset(array=w537, new element=w533, index=w535) -> (w534:T10)
                        n150 = global write "校准数据全局变量.vi" "硅酸盐曲线模型"(w534) -> ()
                      }
                      frame 8 {
                        n151 = case shown="\"空白校准\"" w600 {
                          tunnel: w599 -> [_ w609 w617 w625 w633 w641]
                          tunnel: w598 -> [_ w608 w616 w624 w632 w640]
                          tunnel: w597 -> [_ w607 w615 w623 w631 w639]
                          tunnel: w596 -> [_ w606 w614 w622 w630 w638]
                          tunnel: w595 -> [w601 w604 w612 w620 w628 w636]
                          tunnel: [w601 w603 w611 w619 w627 w635] -> w593
                          tunnel: w594 -> [_ w602 w610 w618 w626 w634]
                          frame "未选择", Default {
                          }
                          frame "空白校准" {
                            n152 = Bundle By Name(cluster=w604, "标液浓度1"=w609, "测量吸光度1"=w608, "模型"=w607, "精度"=w606, "样品1启用"=TRUE, "标样一校准时间"=w602) -> (w603:T6)
                          }
                          frame "标样校准" {
                            n153 = Bundle By Name(cluster=w612, "标液浓度2"=w617, "测量吸光度2"=w616, "模型"=w615, "精度"=w614, "样品2启用"=TRUE ("样品1启用"), "标样二校准时间"=w610) -> (w611:T6)
                          }
                          frame "标样核查" {
                            n154 = Bundle By Name(cluster=w620, "标液浓度3"=w625, "测量吸光度3"=w624, "模型"=w623, "精度"=w622, "样品3启用"=TRUE ("样品1启用"), "标样三校准时间"=w618) -> (w619:T6)
                          }
                          frame "零点核查" {
                            n155 = Bundle By Name(cluster=w628, "标液浓度4"=w633, "测量吸光度4"=w632, "模型"=w631, "精度"=w630, "样品4启用"=TRUE ("样品1启用"), "标样四校准时间"=w626) -> (w627:T6)
                          }
                          frame "跨度核查" {
                            n156 = Bundle By Name(cluster=w636, "标液浓度5"=w641, "测量吸光度5"=w640, "模型"=w639, "精度"=w638, "样品5启用"=TRUE ("样品1启用"), "标样五校准时间"=w634) -> (w635:T6)
                          }
                        }
                        n157 = call "曲线模型计算.vi"("曲线模型"=w593) -> ("输出簇"=w590:T6)  [unwired: 10 in]
                        n158 = global read "校准数据全局变量.vi" "硫化物曲线模型"() -> (w592:T10)
                        n159 = Bundle By Name(cluster=w590, "标定时间"=w587) -> (w588:T6)
                        n160 = Replace Array Subset(array=w592, new element=w588, index=w591) -> (w589:T10)
                        n161 = global write "校准数据全局变量.vi" "硫化物曲线模型"(w589) -> ()
                      }
                      frame 22 {
                        n162 = case shown="\"标样核查\"" w655 {
                          tunnel: w654 -> [_ w664 w672 w680 w688 w696]
                          tunnel: w653 -> [_ w663 w671 w679 w687 w695]
                          tunnel: w652 -> [_ w662 w670 w678 w686 w694]
                          tunnel: w651 -> [_ w661 w669 w677 w685 w693]
                          tunnel: w650 -> [w656 w659 w667 w675 w683 w691]
                          tunnel: [w656 w658 w666 w674 w682 w690] -> w648
                          tunnel: w649 -> [_ w657 w665 w673 w681 w689]
                          frame "未选择", Default {
                          }
                          frame "空白校准" {
                            n163 = Bundle By Name(cluster=w659, "标液浓度1"=w664, "测量吸光度1"=w663, "模型"=w662, "精度"=w661, "样品1启用"=TRUE, "标样一校准时间"=w657) -> (w658:T6)
                          }
                          frame "标样校准" {
                            n164 = Bundle By Name(cluster=w667, "标液浓度2"=w672, "测量吸光度2"=w671, "模型"=w670, "精度"=w669, "样品2启用"=TRUE ("样品1启用"), "标样二校准时间"=w665) -> (w666:T6)
                          }
                          frame "标样核查" {
                            n165 = Bundle By Name(cluster=w675, "标液浓度3"=w680, "测量吸光度3"=w679, "模型"=w678, "精度"=w677, "样品3启用"=TRUE ("样品1启用"), "标样三校准时间"=w673) -> (w674:T6)
                          }
                          frame "零点核查" {
                            n166 = Bundle By Name(cluster=w683, "标液浓度4"=w688, "测量吸光度4"=w687, "模型"=w686, "精度"=w685, "样品4启用"=TRUE ("样品1启用"), "标样四校准时间"=w681) -> (w682:T6)
                          }
                          frame "跨度核查" {
                            n167 = Bundle By Name(cluster=w691, "标液浓度5"=w696, "测量吸光度5"=w695, "模型"=w694, "精度"=w693, "样品5启用"=TRUE ("样品1启用"), "标样五校准时间"=w689) -> (w690:T6)
                          }
                        }
                        n168 = call "曲线模型计算.vi"("曲线模型"=w648) -> ("输出簇"=w646:T6)  [unwired: 10 in]
                        n169 = global read "校准数据全局变量.vi" "CODcr曲线模型"() -> (w647:T10)
                        n170 = Bundle By Name(cluster=w646, "标定时间"=w642) -> (w643:T6)
                        n171 = Replace Array Subset(array=w647, new element=w643, index=w645) -> (w644:T10)
                        n172 = global write "校准数据全局变量.vi" "CODcr曲线模型"(w644) -> ()
                      }
                      frame 21 {
                        n173 = case shown="\"标样核查\"" w710 {
                          tunnel: w709 -> [_ w719 w727 w735 w743 w751]
                          tunnel: w708 -> [_ w718 w726 w734 w742 w750]
                          tunnel: w707 -> [_ w717 w725 w733 w741 w749]
                          tunnel: w706 -> [_ w716 w724 w732 w740 w748]
                          tunnel: w705 -> [w711 w714 w722 w730 w738 w746]
                          tunnel: [w711 w713 w721 w729 w737 w745] -> w703
                          tunnel: w704 -> [_ w712 w720 w728 w736 w744]
                          frame "未选择", Default {
                          }
                          frame "空白校准" {
                            n174 = Bundle By Name(cluster=w714, "标液浓度1"=w719, "测量吸光度1"=w718, "模型"=w717, "精度"=w716, "样品1启用"=TRUE, "标样一校准时间"=w712) -> (w713:T6)
                          }
                          frame "标样校准" {
                            n175 = Bundle By Name(cluster=w722, "标液浓度2"=w727, "测量吸光度2"=w726, "模型"=w725, "精度"=w724, "样品2启用"=TRUE ("样品1启用"), "标样二校准时间"=w720) -> (w721:T6)
                          }
                          frame "标样核查" {
                            n176 = Bundle By Name(cluster=w730, "标液浓度3"=w735, "测量吸光度3"=w734, "模型"=w733, "精度"=w732, "样品3启用"=TRUE ("样品1启用"), "标样三校准时间"=w728) -> (w729:T6)
                          }
                          frame "零点核查" {
                            n177 = Bundle By Name(cluster=w738, "标液浓度4"=w743, "测量吸光度4"=w742, "模型"=w741, "精度"=w740, "样品4启用"=TRUE ("样品1启用"), "标样四校准时间"=w736) -> (w737:T6)
                          }
                          frame "跨度核查" {
                            n178 = Bundle By Name(cluster=w746, "标液浓度5"=w751, "测量吸光度5"=w750, "模型"=w749, "精度"=w748, "样品5启用"=TRUE ("样品1启用"), "标样五校准时间"=w744) -> (w745:T6)
                          }
                        }
                        n179 = global read "校准数据全局变量.vi" "CODMn曲线模型"() -> (w702:T10)
                        n180 = call "曲线模型计算.vi"("曲线模型"=w703) -> ("输出簇"=w701:T6)  [unwired: 10 in]
                        n181 = Bundle By Name(cluster=w701, "标定时间"=w697) -> (w698:T6)
                        n182 = Replace Array Subset(array=w702, new element=w698, index=w700) -> (w699:T10)
                        n183 = global write "校准数据全局变量.vi" "CODMn曲线模型"(w699) -> ()
                      }
                      frame 50 {
                        n184 = case shown="\"标样核查\"" w765 {
                          tunnel: w764 -> [_ w774 w782 w790 w798 w806]
                          tunnel: w763 -> [_ w773 w781 w789 w797 w805]
                          tunnel: w762 -> [_ w772 w780 w788 w796 w804]
                          tunnel: w761 -> [_ w771 w779 w787 w795 w803]
                          tunnel: w760 -> [w766 w769 w777 w785 w793 w801]
                          tunnel: [w766 w768 w776 w784 w792 w800] -> w758
                          tunnel: w759 -> [_ w767 w775 w783 w791 w799]
                          frame "未选择", Default {
                          }
                          frame "空白校准" {
                            n185 = Bundle By Name(cluster=w769, "标液浓度1"=w774, "测量吸光度1"=w773, "模型"=w772, "精度"=w771, "样品1启用"=TRUE, "标样一校准时间"=w767) -> (w768:T6)
                          }
                          frame "标样校准" {
                            n186 = Bundle By Name(cluster=w777, "标液浓度2"=w782, "测量吸光度2"=w781, "模型"=w780, "精度"=w779, "样品2启用"=TRUE ("样品1启用"), "标样二校准时间"=w775) -> (w776:T6)
                          }
                          frame "标样核查" {
                            n187 = Bundle By Name(cluster=w785, "标液浓度3"=w790, "测量吸光度3"=w789, "模型"=w788, "精度"=w787, "样品3启用"=TRUE ("样品1启用"), "标样三校准时间"=w783) -> (w784:T6)
                          }
                          frame "零点核查" {
                            n188 = Bundle By Name(cluster=w793, "标液浓度4"=w798, "测量吸光度4"=w797, "模型"=w796, "精度"=w795, "样品4启用"=TRUE ("样品1启用"), "标样四校准时间"=w791) -> (w792:T6)
                          }
                          frame "跨度核查" {
                            n189 = Bundle By Name(cluster=w801, "标液浓度5"=w806, "测量吸光度5"=w805, "模型"=w804, "精度"=w803, "样品5启用"=TRUE ("样品1启用"), "标样五校准时间"=w799) -> (w800:T6)
                          }
                        }
                        n190 = call "曲线模型计算.vi"("曲线模型"=w758) -> ("输出簇"=w756:T6)  [unwired: 10 in]
                        n191 = global read "校准数据全局变量.vi" "氟化物曲线模型"() -> (w757:T10)
                        n192 = Bundle By Name(cluster=w756, "标定时间"=w752) -> (w753:T6)
                        n193 = Replace Array Subset(array=w757, new element=w753, index=w755) -> (w754:T10)
                        n194 = global write "校准数据全局变量.vi" "氟化物曲线模型"(w754) -> ()
                      }
                    }
                  }
                }
                frame #1 {
                  n195 = global read "总磷总氮断电保存全局变量.vi" "校准条件"() -> (w811:cluster{"线性相关系数":dbl})
                  n196 = Unbundle By Name(w811) -> ("线性相关系数"=w809:dbl)
                  n197 = Unbundle By Name(w812) -> ("r^2"=w810:dbl, "二次方程"=w815:cluster{"c":dbl, "x":dbl, "x^2":dbl})
                  n198 = Greater Or Equal?(x=w810, y=w809) -> (x >= y?=w808:bool)
                  n199 = case shown="False" w808 {
                    tunnel: w815 -> [_ w830]
                    tunnel: w814 -> [w818 w825]
                    tunnel: w813 -> [_ w824]
                    tunnel: w812 -> [_ w823]
                    tunnel: [w816 w822] -> w807
                    frame False {
                      w816 = "校准失败，校准条件未满足" ("日志信息")
                      n200 = call "id参数转换.vi"("id"=w818) -> ("table输出"=w817:string)  [unwired: 9 in, 1 out]
                      n201 = Get Date/Time In Seconds() -> (seconds since 1Jan1904=w821:timestamp)
                      n202 = Bundle By Name(cluster=T3 {"时间标识"=timestamp(0 s since 1904-01-01), "设备"="", "日志信息"="", "流程参数"=""} ("data in"), "时间标识"=w821, "设备"=w817, "日志信息"=w816) -> (w820:T3)
                      n203 = call "总磷总氮操作日志.vi"("data in"=w820) -> ()  [unwired: 10 in, 1 out]
                    }
                    frame True {
                      n204 = Unbundle By Name(w830) -> ("x^2"=w832:dbl, "x"=w833:dbl, "c"=w834:dbl)
                      n205 = Bundle By Name(cluster=cluster{"X^2":dbl, "X":dbl, "b":dbl} {"X^2"=0.0, "X"=0.0, "b"=0.0} ("公式"), "X^2"=w832, "X"=w833, "b"=w834) -> (w826:cluster{"X^2":dbl, "X":dbl, "b":dbl})
                      n206 = for {
                        N: 8 -> [_]
                        shift-right: [w840] -> w827
                        shift-left: errorcluster {"status"=FALSE, "code"=0, "source"=""} ("error out") -> [w838]
                        tunnel: w826 -> [w837]
                        tunnel: w825 -> [w836]
                        tunnel: w824 -> [w835]
                        i -> [w839]
                        n207 = call "公式写入.vi"("公式"=w837, "error in (no error)"=w838, "量程"=w835, "测量模式"=w839, "测量参数"=w836) -> ("error out"=w840:errorcluster)  [unwired: 6 in]
                      }
                      n208 = case shown="Error" w827 {
                        tunnel: w825 -> [w844 _]
                        tunnel: w824 -> [w843 _]
                        tunnel: w823 -> [w842 _]
                        tunnel: ["校准成功" "校准失败，公式写入异常"] -> w822
                        frame No Error {
                          n209 = call "校准记录.vi"("曲线模型"=w842, "量程"=w843, "校准参数"=w844) -> ()  [unwired: 8 in, 1 out]
                        }
                        frame Error {
                        }
                      }
                    }
                  }
                  n210 = global write "VAR总磷总氮全局变量.vi" "校准结果指示"(w807) -> ()
                }
              }
            }
          }
          frame #1 {
            n211 = call "校准数据写入配置文件.vi"() -> ()  [unwired: 11 in, 1 out]
          }
        }
      }
      frame "结束" {
        n212 = Release Notifier(notifier=w853) -> ()  [unwired: 2 in, 3 out]
        n213 = Release Queue(queue=w854) -> ()  [unwired: 2 in, 3 out]
      }
    }
    n214 = Not(x=w12) -> (.not. x?=w13:bool)
    n215 = global write "VAR总磷总氮全局变量.vi" "校准运行状态"(w13) -> ()
    n216 = global write "VAR总磷总氮全局变量.vi" "校准任务"(w10) -> ()
  }
